vi "Motor rated torque.vi"(8 "error in":errorcluster, 11 "Motor Base in":refnum<class "Motor Base.lvclass">) -> (0 "error out":errorcluster, 2 "Data":u32, 3 "Motor Base out":refnum<class "Motor Base.lvclass">)   [LabVIEW 2016, in "Motor Base.lvlib" / "Motor Base.lvclass"]
uses:
  Motor Base.lvclass
  Data Type.ctl
  AccessType.ctl
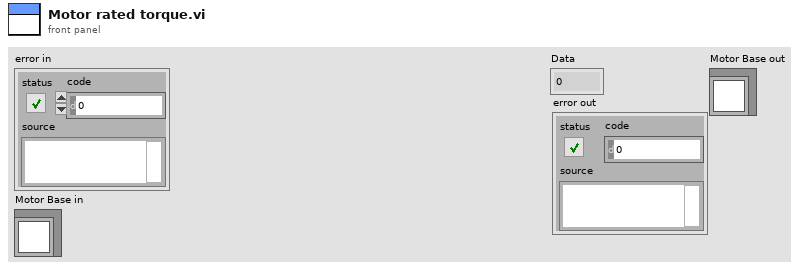
[diagram p1: front panel]
types:
  T1 = typedef "Motor Base.lvlib/Motor Base.lvclass/AccessType.ctl" = enum16{"Write", "Read", "Read Only"}
  T2 = typedef "Motor Base.lvlib/Motor Base.lvclass/Data Type.ctl" = enum16{"BOOL", "I16", "I32", "I8", "OS", "U16", "U32", "U8", "VS"}
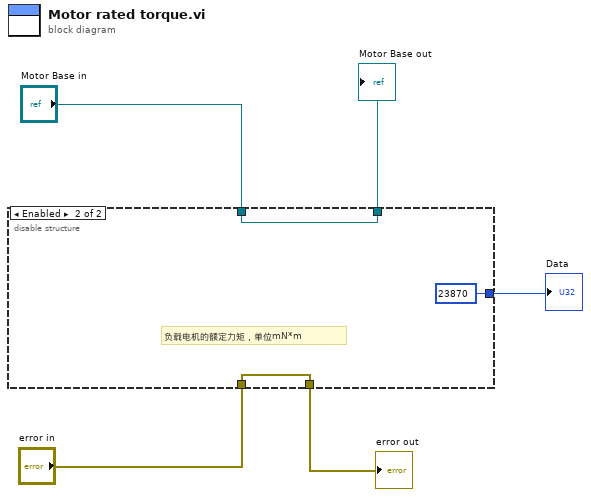
[diagram p0: block diagram]
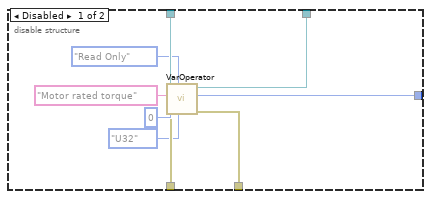
[diagram p2: hidden frame]
diagram:
  n1 = disable-structure shown="Enabled" {
    disable-tunnel: "error in" -> [w12 w16]
    disable-tunnel: [w11 w16] -> w4
    disable-tunnel: "Motor Base in" -> [w10 w17]
    disable-tunnel: [w9 w17] -> w2
    disable-tunnel: [w6 u32 23870 ("Data")] -> w1
    frame Disabled {
      n2 = call-dynamic "VarOperator.vi"("Data Type"=Data_Type."U32", "ro/w/r"=AccessType."Read Only", "error in"=w12, "Data"=i64 0, "PDO Name"="Motor rated torque", "Motor Base in"=w10) -> ("error out"=w11:errorcluster, "Data"=w6:i64, "Motor Base out"=w9:refnum<class "Motor Base.lvclass">)  [unwired: 1 in, 2 out]
    }
    frame Enabled {
      # "负载电机的额定力矩，单位mN*m"
    }
  }
  "error out" <- w4
  "Motor Base out" <- w2
  "Data" <- w1
